vi "Matlab_toGage.vi"(6 "streaming":bool, 8 "Xmax":dbl format="%#_13g", 9 "Zmax":dbl format="%#_13g", 10 "X0":dbl format="%#_13g", 11 "Sample Rate":dbl) -> (0 "Acquisition  parameters out":T1={"Sample Rate"=1000000.0, "Clock mode"=enum."Internal", "Mode"=0, "post trigger"=8192.0, "Segment Size"=8192.0, "Trigger Timeout"=100000.0, "Trigger Holdoff"=0.0, "Trigger Delay"=0.0, "number of records"=5} {"Mode" items=["Single", "Dual", "Quad", "Octal"]})   [LabVIEW 2015]
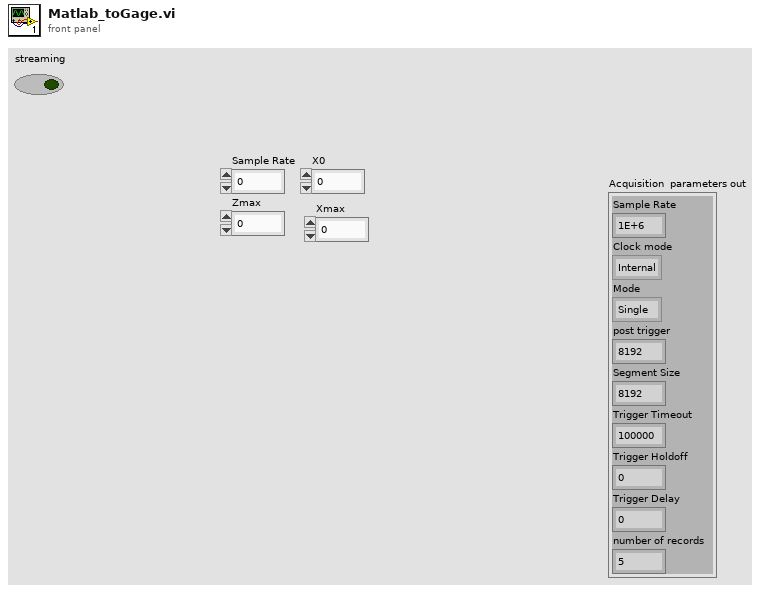
[diagram p1: front panel]
types:
  T1 = cluster{"Sample Rate":dbl, "Clock mode":enum16{"Internal", "External", "Reference"}, "Mode":u16, "post trigger":dbl, "Segment Size":dbl, "Trigger Timeout":dbl, "Trigger Holdoff":dbl, "Trigger Delay":dbl, "number of records":u32}
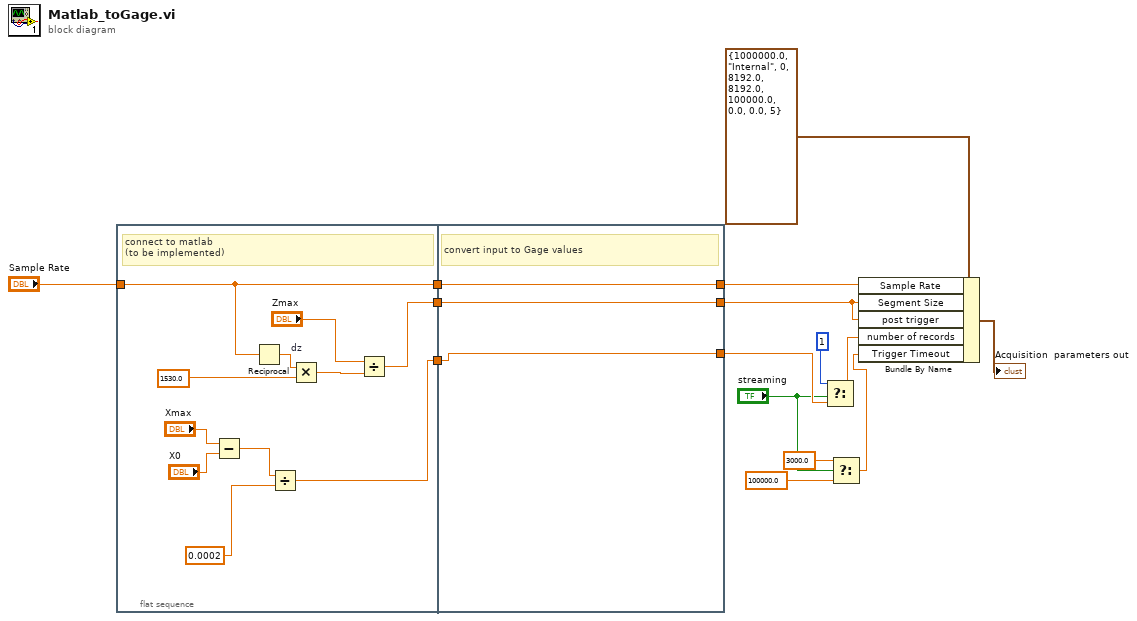
[diagram p0: block diagram]
diagram:
  n1 = flat-sequence {
    tunnel: "Sample Rate" -> [w26]
    tunnel: [w26] -> w12
    tunnel: [w21] -> w10
    tunnel: [w16] -> w9
    tunnel: w12 -> [w29]
    tunnel: [w29] -> w11
    tunnel: w10 -> [w28]
    tunnel: [w28] -> w8
    tunnel: w9 -> [w27]
    tunnel: [w27] -> w7
    frame #0 {
      # "connect to matlab\n(to be implemented)"
      n2 = Subtract(x="Xmax", y="X0") -> (x-y=w18:dbl)
      n3 = Reciprocal(x=w26) -> (1/x=w25:dbl)
      n4 = Divide(x=w18, y=0.0002) -> (x/y=w16:dbl)
      n5 = Multiply "dz"(x=w25, y=1530.0) -> (x*y=w23:dbl)
      n6 = Divide(x="Zmax", y=w23) -> (x/y=w21:dbl)
    }
    frame #1 {
      # "convert input to Gage values"
    }
  }
  n7 = Select(t=1, s="streaming", f=w7) -> (s? t:f=w5:dbl)
  n8 = Select(t=3000.0, s="streaming", f=100000.0 ("Trigger Timeout")) -> (s? t:f=w1:dbl)
  n9 = Bundle By Name(cluster=T1 {"Sample Rate"=1000000.0, "Clock mode"=enum."Internal", "Mode"=0, "post trigger"=8192.0, "Segment Size"=8192.0, "Trigger Timeout"=100000.0, "Trigger Holdoff"=0.0, "Trigger Delay"=0.0, "number of records"=5} ("Acquisition  parameters out"), "Sample Rate"=w11, "Segment Size"=w8, "post trigger"=w8, "number of records"=w5, "Trigger Timeout"=w1) -> (→"Acquisition  parameters out":T1)
